vi "Initialize All Actor.vi"(8 "error in (no error)":errorcluster, 10 "Actor Queues":T1, 11 "Supervisor in":refnum<class "Supervisor.lvclass">) -> (0 "error out":errorcluster, 3 "Supervisor out":refnum<class "Supervisor.lvclass">)   [LabVIEW 2020, in "Supervisor.lvlib" / "Supervisor.lvclass"]
uses:
  Supervisor.lvclass
  Supervisor.lvclass/Supervisor.ctl
  DAQ DI/DAQ DI Messages/Initialize DAQ Channel Msg/Initialize DAQ Channel Msg.lvclass
  DAQ AI/DAQ AI Messages/Initialize DAQ Channel Msg/Initialize DAQ Channel Msg.lvclass
  UI/UI Messages/Initialize Msg/Initialize Msg.lvclass
  <vilib>/Utility/file.llb/Read Delimited Spreadsheet (string).vi
  <vilib>/ActorFramework/Message Enqueuer/Message Enqueuer.lvclass
  TypeDef/Actor Queues.ctl
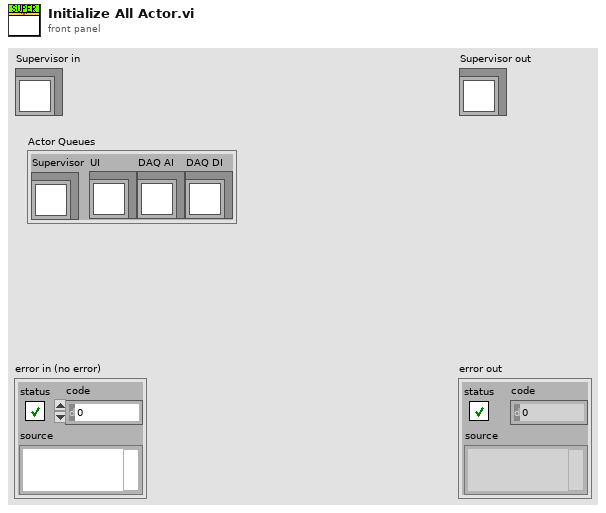
[diagram p1: front panel]
types:
  T1 = typedef "Supervisor.lvlib/Supervisor.lvclass/Actor Queues.ctl" = cluster{"Supervisor":refnum<class "Message Enqueuer.lvclass">, "UI":refnum<class "Message Enqueuer.lvclass">, "DAQ AI":refnum<class "Message Enqueuer.lvclass">, "DAQ DI":refnum<class "Message Enqueuer.lvclass">}
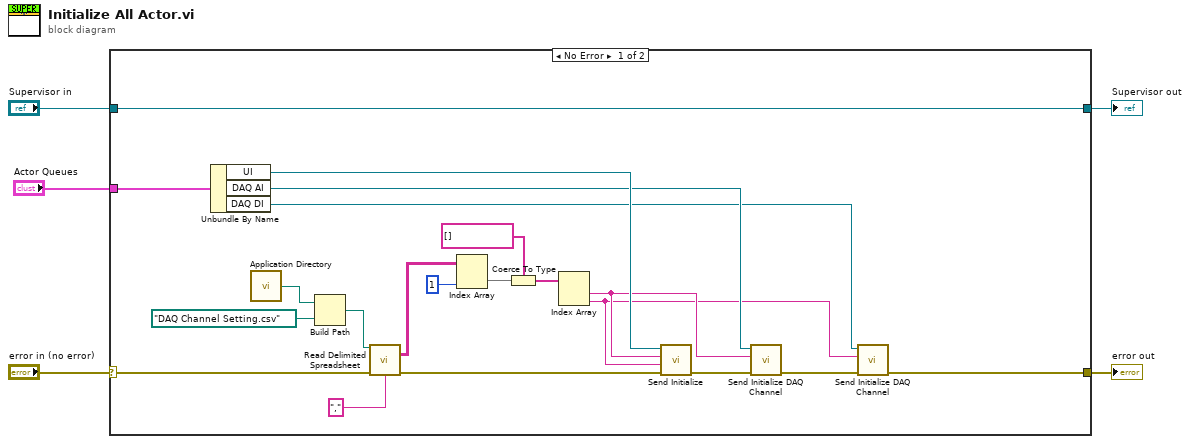
[diagram p0: block diagram]
diagram:
  n1 = case shown="No Error" "error in (no error)" {
    selector: "error in (no error)" -> [w18 w28]
    tunnel: [w19 w28] -> w4
    tunnel: [w26 w27] -> w2
    tunnel: "Supervisor in" -> [w26 w27]
    tunnel: "Actor Queues" -> [w25 _]
    frame No Error {
      n2 = Unbundle By Name(w25) -> ("UI"=w24:refnum<class "Message Enqueuer.lvclass">, "DAQ AI"=w23:refnum<class "Message Enqueuer.lvclass">, "DAQ DI"=w22:refnum<class "Message Enqueuer.lvclass">)
      n3 = call <vilib>:"Application Directory.vi"() -> ("Application Directory"=w17:path)
      n4 = Build Path(base path=w17, name or relative path=path "DAQ Channel Setting.csv") -> (appended path=w15:path)
      n5 = call-poly <vilib>:"Read Delimited Spreadsheet.vi"("file path (dialog if empty)"=w15, "error in (no error)"=w18, "delimiter (\\t)"="," ("delimiter (\\t)")) -> ("all rows"=w14:string[][], "error out"=w9:errorcluster)  [unwired: 7 in, 4 out]
      n6 = Index Array(array=w14, index (col)=1 ("disabled index (col)")) -> (element=w11:string[])  [unwired: 1 in]
      n7 = Coerce To Type(0:w11, 1:tag[] [] ("DAQmx Analog Channel")) -> (2:w10:tag[])
      n8 = Index Array(array=w10) -> (element #1=w8:tag, element #2=w7:tag)  [unwired: 2 in]
      n9 = call "Send Initialize.vi"("error in (no error)"=w9, "DAQmx Digital Channel"=w7, "DAQmx Analog Channel"=w8, "Message Enqueuer"=w24) -> ("error out"=w20:errorcluster)  [unwired: 6 in, 1 out]
      n10 = call "Send Initialize DAQ Channel.vi"("error in (no error)"=w20, "DAQmx Analog Channel"=w8, "Message Enqueuer"=w23) -> ("error out"=w21:errorcluster)  [unwired: 7 in, 1 out]
      n11 = call "Send Initialize DAQ Channel.vi"("error in (no error)"=w21, "DAQmx Digital Channel"=w7, "Message Enqueuer"=w22) -> ("error out"=w19:errorcluster)  [unwired: 7 in, 1 out]
    }
    frame Error {
    }
  }
  "error out" <- w4
  "Supervisor out" <- w2
